vi "PIDDirection.vi"(1 "LoadCellIn":dbl[](array[numeric]), 2 "SetPointIn":dbl[](array[numeric])) -> (0 "MotorDirOut":bool[](array[boolean]))   [LabVIEW 2013]
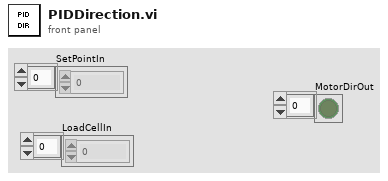
[diagram p1: front panel]
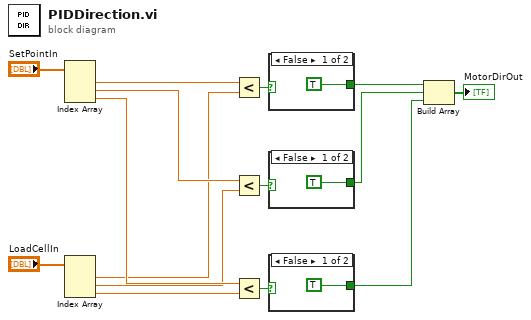
[diagram p0: block diagram]
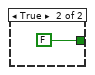
[diagram p2: hidden frame]
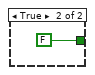
[diagram p3: hidden frame]
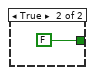
[diagram p4: hidden frame]
diagram:
  n1 = Index Array(array="SetPointIn") -> (element #1=w12:dbl, element #2=w11:dbl, element #3=w10:dbl)  [unwired: 3 in]
  n2 = Index Array(array="LoadCellIn") -> (element #1=w5:dbl, element #2=w6:dbl, element #3=w7:dbl)  [unwired: 3 in]
  n3 = Less?(x=w12, y=w5) -> (x < y?=w15:bool)
  n4 = Less?(x=w11, y=w6) -> (x < y?=w14:bool)
  n5 = Less?(x=w10, y=w7) -> (x < y?=w13:bool)
  n6 = case shown="False" w15 {
    tunnel: [TRUE FALSE] -> w4
    frame False {
    }
    frame True {
    }
  }
  n7 = case shown="False" w14 {
    tunnel: [TRUE FALSE] -> w3
    frame False {
    }
    frame True {
    }
  }
  n8 = case shown="False" w13 {
    tunnel: [TRUE FALSE] -> w2
    frame False {
    }
    frame True {
    }
  }
  n9 = Build Array(w4, w3, w2) -> (→"MotorDirOut":bool[])
